vi "handleIncomingMessages.vi"(8 "error in (no error)":errorcluster, 11 "DataListenerThisComponent in":refnum<class "DataListenerThisComponent.lvclass">) -> (0 "error out":errorcluster, 3 "DataListenerThisComponent out":refnum<class "DataListenerThisComponent.lvclass">)   [LabVIEW 2016, in "DataListenerThisComponent.lvclass"]
uses:
  DataListenerThisComponent.lvclass
  home/andres/ct_cmpuserevents/ComponentTemplateCore/ComponentModel/ComponentModel/DataListener/DataListener.lvclass
  ComponentTemplateCore/ComponentModel/ComponentModel/DataListener/DataListener.lvclass/DataListener.ctl
  DataListenerThisComponent.lvclass/DataListenerThisComponent.ctl
  PubSubDataEvent/PubSubDataEvent.lvclass/PubSubDataEvent.ctl
  Typedefs/CommandValue.ctl
  ComponentTemplateCore/ComponentModel/ComponentModel/DataListenerGlobals/stop.vi
  ICommandFactory/ICommandFactory.lvclass
  Typedefs/EXATypedefs.lvlib
  ComponentTemplateCore/ComponentModel/ComponentModel/DataListener/DataListener.lvclass
  ComponentTemplateCore/ComponentModel/ComponentModel/DataListenerGlobals/DataListenerGlobals.lvlib
  PubSubDataEvent/PubSubDataEvent.lvclass
  ComponentTemplateCore/ComponentModel/ComponentModel/Rendezvous/Rendezvous.lvclass
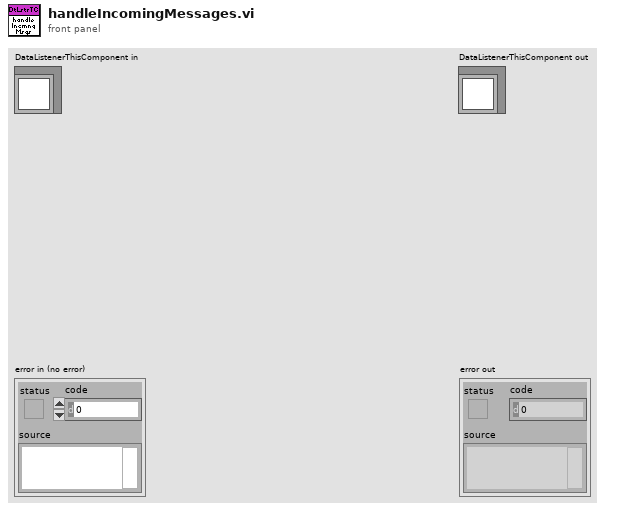
[diagram p1: front panel]
types:
  T1 = typedef "EXATypedefs.lvlib/SubDataEvents.ctl" = cluster{"ClearError":refnum<user-event>, "Disable":refnum<user-event>, "Enable":refnum<user-event>, "Exit":refnum<user-event>, "GoToStandby":refnum<user-event>, "HeartbeatIn":refnum<user-event>, "Start":refnum<user-event>}
  T2 = typedef "EXATypedefs.lvlib/CommandValue.ctl" = enum16{"ClearError", "Disable", "Enable", "Exit", "GoToStandby", "OnHeartbeat", "OnIncomingMessagingError", "OnInterrupt", "Start"}
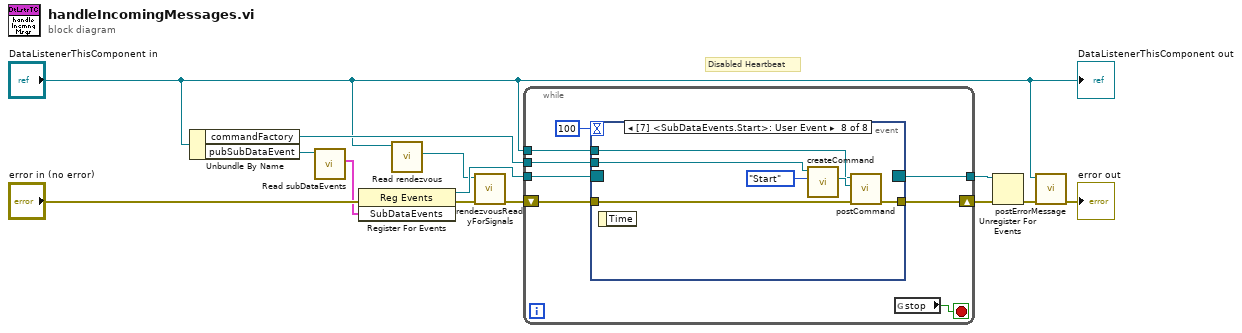
[diagram p0: block diagram]
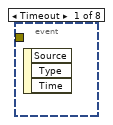
[diagram p2: hidden frame]
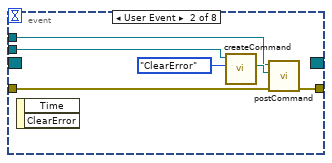
[diagram p3: hidden frame]
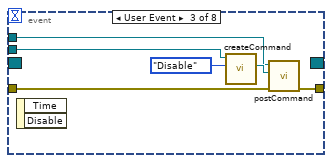
[diagram p4: hidden frame]
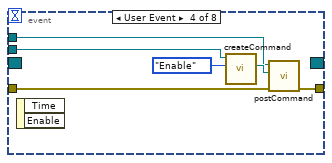
[diagram p5: hidden frame]
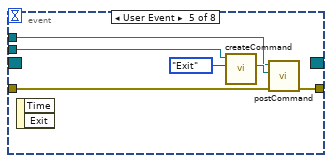
[diagram p6: hidden frame]
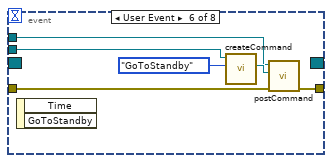
[diagram p7: hidden frame]
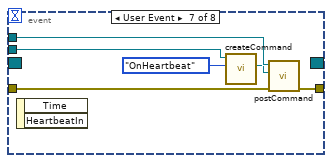
[diagram p8: hidden frame]
diagram:
  # "Disabled Heartbeat"
  n1 = Unbundle By Name("DataListenerThisComponent in") -> ("commandFactory"=w13:refnum<class "ICommandFactory.lvclass">, "pubSubDataEvent"=w6:refnum<class "PubSubDataEvent.lvclass">)
  n2 = call "Read subDataEvents.vi"("PubSubDataEvent in"=w6) -> ("SubDataEvents"=w5:T1)  [unwired: 9 in, 1 out]
  n3 = register-events(error in="error in (no error)", w5) -> (reference out=w9:refnum<event-registration>, error out=w2:errorcluster)  [unwired: 1 in]
  n4 = call "Read rendezvous.vi"("DataListener in"="DataListenerThisComponent in") -> ("rendezvous"=w3:refnum<class "Rendezvous.lvclass">)  [unwired: 9 in, 1 out]
  n5 = call "rendezvousReadyForSignals.vi"("error in (no error)"=w2, "Rendezvous in"=w3) -> ("error out"=w1:errorcluster)  [unwired: 8 in, 1 out]
  n6 = while {
    tunnel: w9 -> [w21]
    tunnel: [w20] -> w10
    tunnel: w13 -> [w19]
    tunnel: "DataListenerThisComponent in" -> [w18]
    shift-right: [w16] -> w12
    shift-left: w1 -> [w17]
    stop <- w15 stop-if-true
    n7 = event shown="[7] <SubDataEvents.Start>: User Event" {
      selector: w21 -> [_ _ _ _ _ _ _ _]
      dyn-events: [_ _ _ _ _ _ _ _] -> w20
      timeout: 100 -> [_ _ _ _ _ _ _ _]
      tunnel: w19 -> [_ w26 w32 w38 w44 w50 w57 w62]
      tunnel: w18 -> [_ w24 w30 w36 w42 w48 w56 w60]
      tunnel: w17 -> [_ w23 w29 w35 w41 w47 w55 w59]
      tunnel: [_ w22 w28 w34 w40 w46 w54 w58] -> w16
      event Timeout {
        n8 = event-data() -> ()  [unwired: 1 in, 3 out]
      }
      event User Event {
        n9 = event-data() -> ()  [unwired: 1 in, 2 out]
        n10 = call-dynamic "createCommand.vi"("commandValue"=CommandValue."ClearError", "ICommandFactory in"=w26) -> ("command"=w25:refnum<class "Command.lvclass">)  [unwired: 7 in, 2 out]
        n11 = call "postCommand.vi"("error in (no error)"=w23, "command"=w25, "DataListener in"=w24) -> ("error out"=w22:errorcluster)  [unwired: 7 in, 1 out]
      }
      event User Event {
        n12 = event-data() -> ()  [unwired: 1 in, 2 out]
        n13 = call-dynamic "createCommand.vi"("commandValue"=CommandValue."Disable", "ICommandFactory in"=w32) -> ("command"=w31:refnum<class "Command.lvclass">)  [unwired: 7 in, 2 out]
        n14 = call "postCommand.vi"("error in (no error)"=w29, "command"=w31, "DataListener in"=w30) -> ("error out"=w28:errorcluster)  [unwired: 7 in, 1 out]
      }
      event User Event {
        n15 = event-data() -> ()  [unwired: 1 in, 2 out]
        n16 = call-dynamic "createCommand.vi"("commandValue"=CommandValue."Enable", "ICommandFactory in"=w38) -> ("command"=w37:refnum<class "Command.lvclass">)  [unwired: 7 in, 2 out]
        n17 = call "postCommand.vi"("error in (no error)"=w35, "command"=w37, "DataListener in"=w36) -> ("error out"=w34:errorcluster)  [unwired: 7 in, 1 out]
      }
      event User Event {
        n18 = event-data() -> ()  [unwired: 1 in, 2 out]
        n19 = call-dynamic "createCommand.vi"("commandValue"=CommandValue."Exit", "ICommandFactory in"=w44) -> ("command"=w43:refnum<class "Command.lvclass">)  [unwired: 7 in, 2 out]
        n20 = call "postCommand.vi"("error in (no error)"=w41, "command"=w43, "DataListener in"=w42) -> ("error out"=w40:errorcluster)  [unwired: 7 in, 1 out]
      }
      event User Event {
        n21 = event-data() -> ()  [unwired: 1 in, 2 out]
        n22 = call-dynamic "createCommand.vi"("commandValue"=CommandValue."GoToStandby", "ICommandFactory in"=w50) -> ("command"=w49:refnum<class "Command.lvclass">)  [unwired: 7 in, 2 out]
        n23 = call "postCommand.vi"("error in (no error)"=w47, "command"=w49, "DataListener in"=w48) -> ("error out"=w46:errorcluster)  [unwired: 7 in, 1 out]
      }
      event User Event {
        n24 = event-data() -> ()  [unwired: 1 in, 2 out]
        n25 = call-dynamic "createCommand.vi"("commandValue"=CommandValue."OnHeartbeat", "ICommandFactory in"=w57) -> ("command"=w52:refnum<class "Command.lvclass">)  [unwired: 7 in, 2 out]
        n26 = call "postCommand.vi"("error in (no error)"=w55, "command"=w52, "DataListener in"=w56) -> ("error out"=w54:errorcluster)  [unwired: 7 in, 1 out]
      }
      event User Event {
        n27 = event-data() -> ()  [unwired: 1 in, 1 out]
        n28 = call-dynamic "createCommand.vi"("commandValue"=CommandValue."Start", "ICommandFactory in"=w62) -> ("command"=w61:refnum<class "Command.lvclass">)  [unwired: 7 in, 2 out]
        n29 = call "postCommand.vi"("error in (no error)"=w59, "command"=w61, "DataListener in"=w60) -> ("error out"=w58:errorcluster)  [unwired: 7 in, 1 out]
      }
    }
    n30 = global read "stop.vi" "stop"() -> (w15:bool)
  }
  n31 = Unregister For Events(event registration refnum=w10, error in=w12) -> (error out=w8:errorcluster)
  n32 = call "postErrorMessage.vi"("error in (no error)"=w8, "DataListener in"="DataListenerThisComponent in") -> ("error out"=→"error out":errorcluster)  [unwired: 8 in, 1 out]
  "DataListenerThisComponent out" <- "DataListenerThisComponent in"
